vi "DAQ Create LINE 0.vi"(3 "error in":errorcluster, 5 "Puerto":dbl) -> (0 "error out":errorcluster, 2 "task out":refnum<k21>)   [LabVIEW 2023]
uses:
  <vilib>/DAQmx/create/channels.llb/DAQmx Create Channel (DO-Digital Output).vi
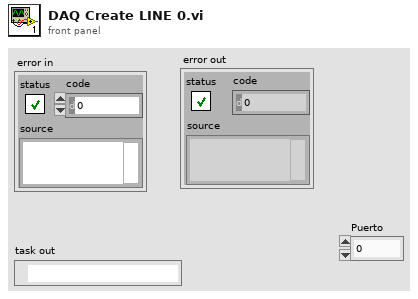
[diagram p1: front panel]
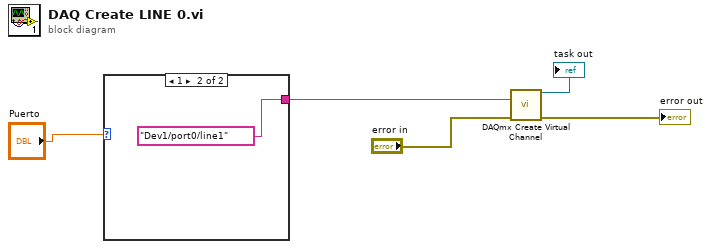
[diagram p0: block diagram]
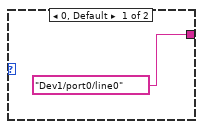
[diagram p2: hidden frame]
diagram:
  n1 = case shown="1" "Puerto" {
    tunnel: [tag "Dev1/port0/line0" ("lines") tag "Dev1/port0/line1" ("lines")] -> w1
    frame 0, Default {
    }
    frame 1 {
    }
  }
  n2 = call-poly <vilib>:"DAQmx Create Virtual Channel.vi"("lines"=w1, "error in"="error in") -> ("task out"=→"task out":refnum<k21>, "error out"=→"error out":errorcluster)  [unwired: 12 in]
